vi "Read States.vi"(8 "error in (no error)":errorcluster, 11 "GoToBallPlacementAllyTactic in":refnum<class "GoToBallPlacementAllyTactic.lvclass">) -> (0 "error out":errorcluster, 2 "States":T1, 3 "GoToBallPlacementAllyTactic out":refnum<class "GoToBallPlacementAllyTactic.lvclass">)   [LabVIEW 2021, in "GoToBallPlacementAllyTactic.lvclass"]
uses:
  GoToBallPlacementAllyTactic.lvclass
  StatesGoToBallPlacementAllyTactic.ctl
  GoToBallPlacementAllyTactic.lvclass/GoToBallPlacementAllyTactic.ctl
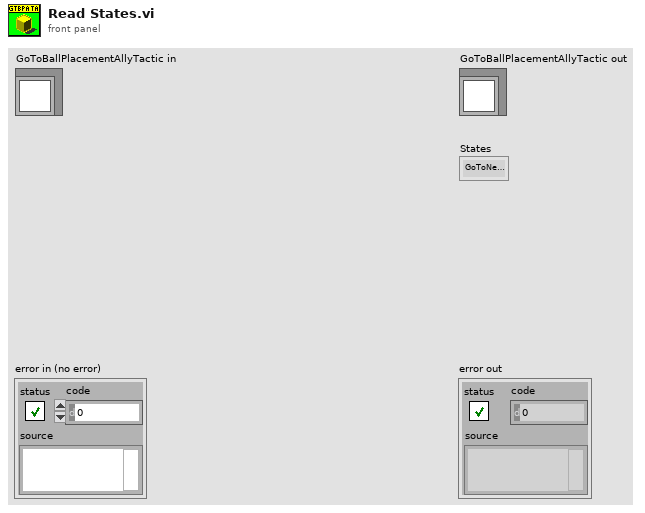
[diagram p1: front panel]
types:
  T1 = typedef "StatesGoToBallPlacementAllyTactic.ctl" = enum16{"GoToNearBall", "GoToBall", "PrepareToPositionBall", "Exit"}
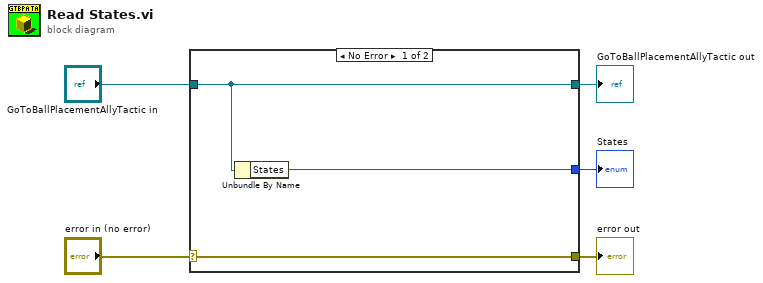
[diagram p0: block diagram]
diagram:
  n1 = case shown="No Error" "error in (no error)" {
    selector: "error in (no error)" -> [w8 w9]
    tunnel: [w8 w9] -> w4
    tunnel: [w7 w10] -> w2
    tunnel: "GoToBallPlacementAllyTactic in" -> [w7 w10]
    tunnel: [w6 _] -> w1
    frame No Error {
      n2 = Unbundle By Name(w7) -> ("States"=w6:T1)
    }
    frame Error {
    }
  }
  "error out" <- w4
  "GoToBallPlacementAllyTactic out" <- w2
  "States" <- w1
